vi "Insert SharedString.vi"(8 "error in":errorcluster, 10 "Value":string, 11 "SharedStringTablePart in":refnum<k24>) -> (0 "error out":errorcluster, 2 "Index":i32, 3 "SharedStringTablePart out":refnum<k24>)   [LabVIEW 2021, in "Open Xml.lvlib"]
uses:
  Open Xml.lvlib
  D:/git/Open-Xml-LabVIEW/dll/DocumentFormat.OpenXml.dll
  dll/DocumentFormat.OpenXml.dll
  D:/git/Open-Xml-LabVIEW/dll/DocumentFormat.OpenXml.Framework.dll
  dll/DocumentFormat.OpenXml.Framework.dll
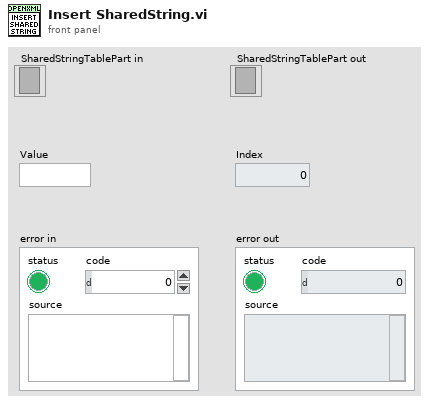
[diagram p1: front panel]
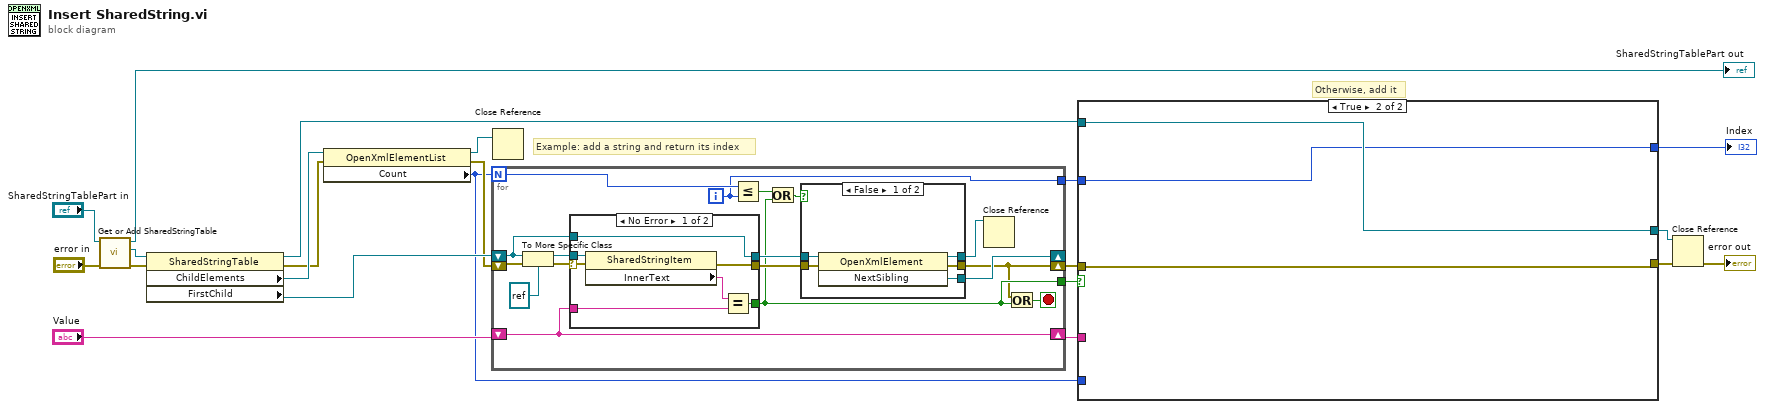
[diagram p0: block diagram]
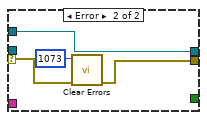
[diagram p2: hidden frame]
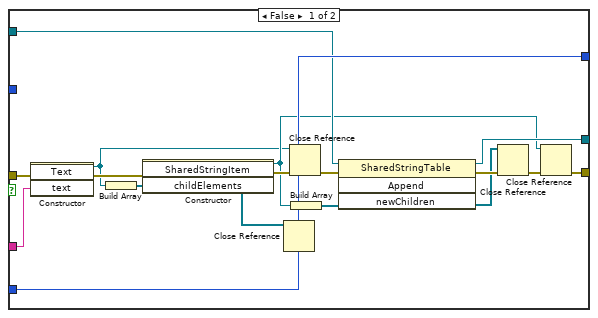
[diagram p4: hidden frame]
diagram:
  # "Otherwise, add it"
  # "Example: add a string and return its index"
  n1 = call "Get or Add SharedStringTable.vi"("error in"="error in", "SharedStringTablePart in"="SharedStringTablePart in") -> ("error out"=w17:errorcluster, "SharedStringTable"=w18:refnum<k24>, "SharedStringTablePart out"=→"SharedStringTablePart out":refnum<k24>)  [unwired: 7 in]
  n2 = property class="SharedStringTable"(reference=w18, error in=w17) -> (reference out=w10:refnum<k24>, error out=w14:errorcluster, "ChildElements"=w19:refnum<k24>, "FirstChild"=w20:refnum<k24>)
  n3 = property class="OpenXmlElementList"(reference=w19, error in=w14) -> (reference out=w12:refnum<k24>, error out=w6:errorcluster, "Count"=w5:i32)
  n4 = for {
    N: w5 -> [w24]
    tunnel: [w25] -> w13
    shift-right: [w22] -> w7
    shift-left: w6 -> [w36]
    shift-right: [w29] -> _
    shift-left: w20 -> [w34]
    tunnel: [w23] -> w4
    shift-right: [w33] -> w9
    shift-left: "Value" -> [w33]
    i -> [w23]
    stop <- w31 stop-if-true
    n5 = To More Specific Class(target class=refnum<k24> refnum ("SharedStringItem"), reference=w34, error in=w36) -> (specific class reference=w38:refnum<k24>, error out=w35:errorcluster)
    n6 = case shown="No Error" w35 {
      selector: w35 -> [w43 w49]
      tunnel: [w41 _] -> w25
      tunnel: w38 -> [w44 _]
      tunnel: w34 -> [w40 w47]
      tunnel: w33 -> [w42 _]
      tunnel: [w39 w46] -> w32
      tunnel: [w40 w47] -> w30
      frame No Error {
        n7 = property class="SharedStringItem"(reference=w44, error in=w43) -> (error out=w39:errorcluster, "InnerText"=w45:string)  [unwired: 1 out]
        n8 = Equal?(x=w45, y=w42) -> (x = y?=w41:bool)
      }
      frame Error {
        n9 = call <vilib>:"Clear Errors.vi"("error in (no error)"=w49, "specific error code to clear (0: all)"=1073) -> ("error out"=w46:errorcluster)  [unwired: 4 in, 1 out]
      }
    }
    n10 = Less Or Equal?(x=w24, y=w23) -> (x <= y?=w27:bool)
    n11 = Or(x=w27, y=w25) -> (x .or. y?=w26:bool)
    n12 = case shown="False" w26 {
      tunnel: w32 -> [w54 w56]
      tunnel: w30 -> [w53 w55]
      tunnel: [w52 _] -> w29
      tunnel: [w51 w56] -> w22
      tunnel: [w50 w55] -> w28
      frame False {
        n13 = invoke class="OpenXmlElement" method="NextSibling"(reference=w53, error in=w54) -> (reference out=w50:refnum<k24>, error out=w51:errorcluster, "NextSibling"=w52:refnum<k24>)  [unwired: 1 in]
      }
      frame True {
      }
    }
    n14 = Close Reference(reference=w28) -> ()  [unwired: 1 in, 1 out]
    n15 = Or(x=w22, y=w25) -> (x .or. y?=w31:bool)
  }
  n16 = Close Reference(reference=w12) -> ()  [unwired: 1 in, 1 out]
  n17 = case shown="True" w13 {
    tunnel: w5 -> [w73 _]
    tunnel: [w73 w75] -> w11
    tunnel: w10 -> [w72 w76]
    tunnel: w9 -> [w64 _]
    tunnel: [w69 w76] -> w3
    tunnel: [w57 w74] -> w8
    tunnel: w4 -> [_ w75]
    tunnel: w7 -> [w60 w74]
    frame False {
      n18 = constructor class="Text"(error in=w60, "text"=w64) -> (reference out=w58:refnum<k24>, error out=w63:errorcluster)  [unwired: 2 in, 2 out]
      n19 = Build Array(w58) -> (w66:refnum<k24>[])
      n20 = constructor class="SharedStringItem"(error in=w63, "childElements"=w66) -> (reference out=w62:refnum<k24>, error out=w65:errorcluster, "childElements"=w61:refnum<k24>[])  [unwired: 2 in, 1 out]
      n21 = Close Reference(reference=w61) -> ()  [unwired: 1 in, 1 out]
      n22 = Close Reference(reference=w58, error in (no error)=w65) -> (error out=w59:errorcluster)
      n23 = Build Array(w62) -> (w67:refnum<k24>[])
      n24 = invoke class="SharedStringTable" method="Append"(reference=w72, error in=w59, "newChildren"=w67) -> (reference out=w69:refnum<k24>, error out=w71:errorcluster, "newChildren"=w68:refnum<k24>[])  [unwired: 1 in, 1 out]
      n25 = Close Reference(reference=w68, error in (no error)=w71) -> (error out=w70:errorcluster)
      n26 = Close Reference(reference=w62, error in (no error)=w70) -> (error out=w57:errorcluster)
    }
    frame True {
    }
  }
  "Index" <- w11
  n27 = Close Reference(reference=w3, error in (no error)=w8) -> (error out=→"error out":errorcluster)
